vi "ManageDrive.vi"(8 "error in (no error)":errorcluster, 11 "config":T1) -> (0 "error out":errorcluster, 1 "free disk space":dbl, 2 "streams deleted":i32, 3 "files deleted":i32)   [LabVIEW 2017, in "FileManager.lvlib"]
uses:
  <vilib>/addons/InsightCM/Devices/Shared/Common/FileManager/FileManager.lvlib
  <vilib>/addons/InsightCM/Devices/Shared/Common/FileManager/controls/config.ctl
panel:
  out "config out":T1
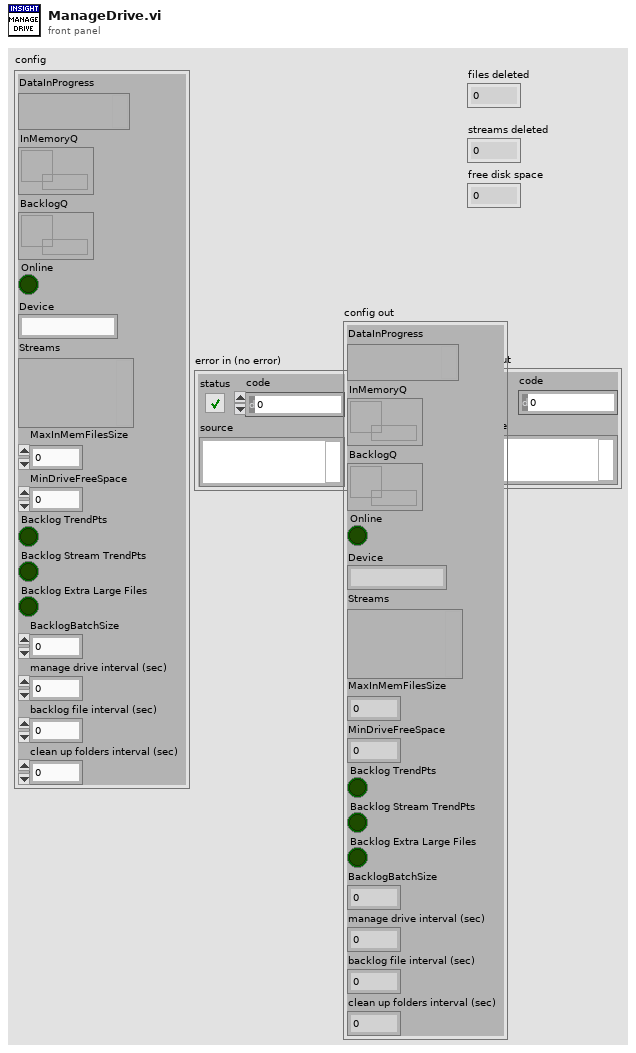
[diagram p1: front panel]
types:
  T1 = typedef "FileManager.lvlib/config.ctl" = cluster{"DataInProgress":variant, "InMemoryQ":refnum<queue>, "BacklogQ":refnum<queue>, "Online":bool, "Device":string, "Streams":variant, "MaxInMemFilesSize":i32, "MinDriveFreeSpace":i32, "Backlog TrendPts":bool, "Backlog Stream TrendPts":bool, "Backlog Extra Large Files":bool, "BacklogBatchSize":i32, "manage drive interval (sec)":dbl, "backlog file interval (sec)":dbl, "clean up folders interval (sec)":dbl}
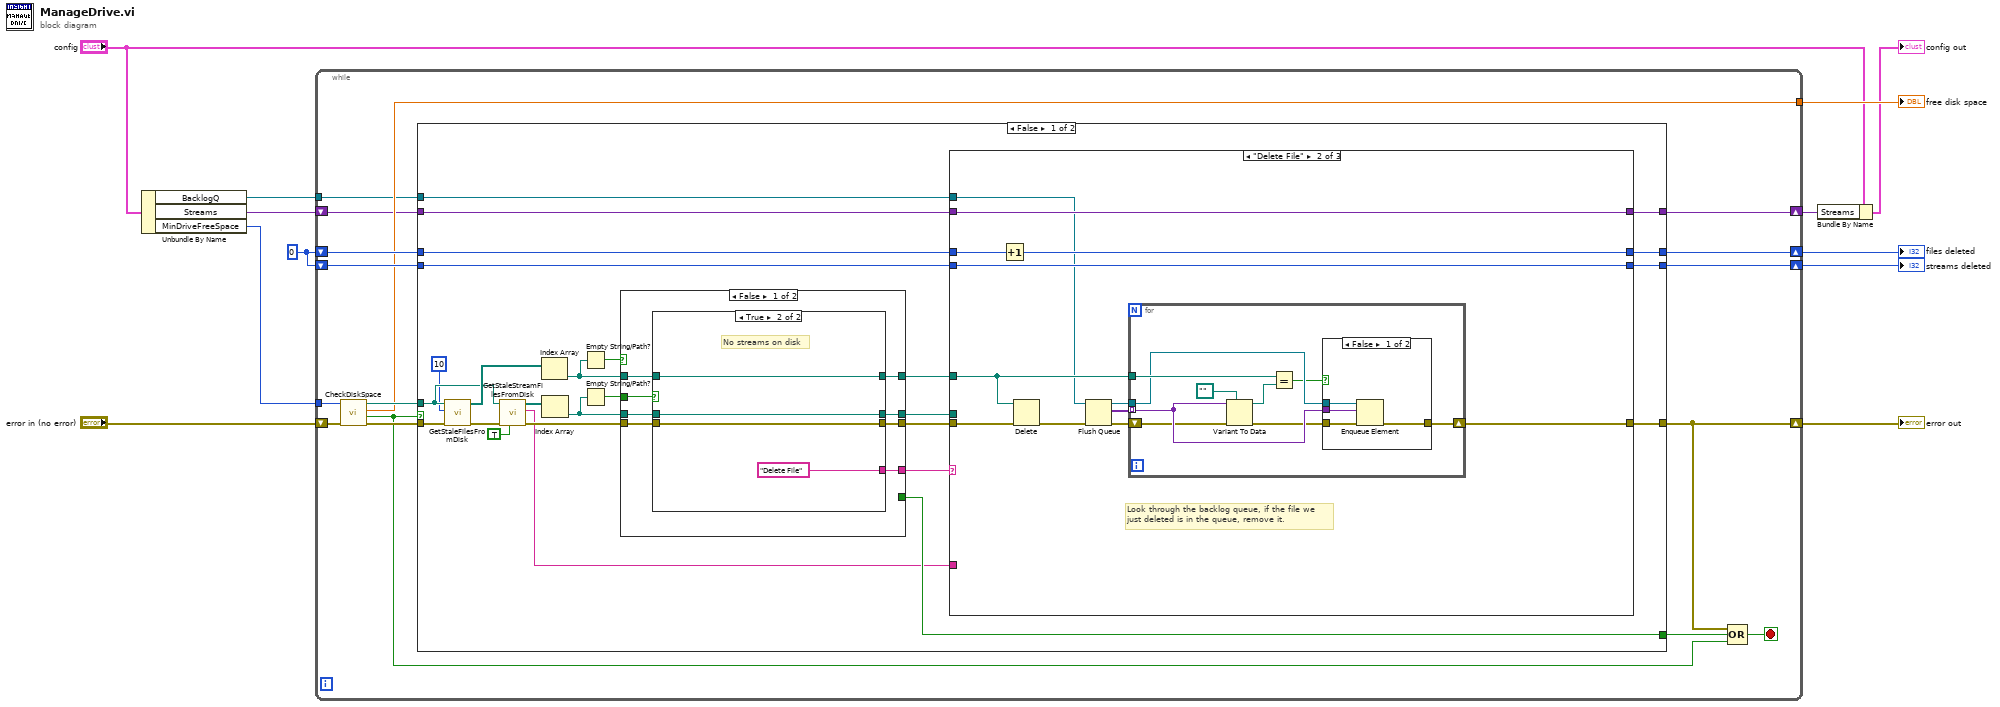
[diagram p0: block diagram]
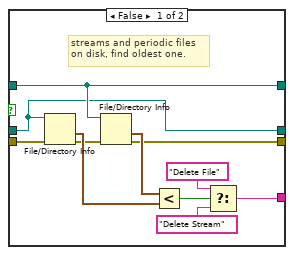
[diagram p2: hidden frame]
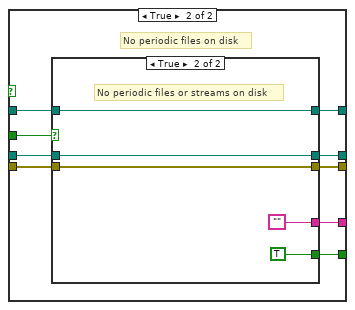
[diagram p3: hidden frame]
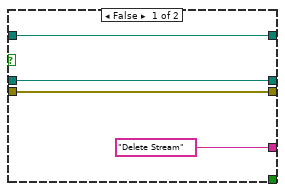
[diagram p4: hidden frame]
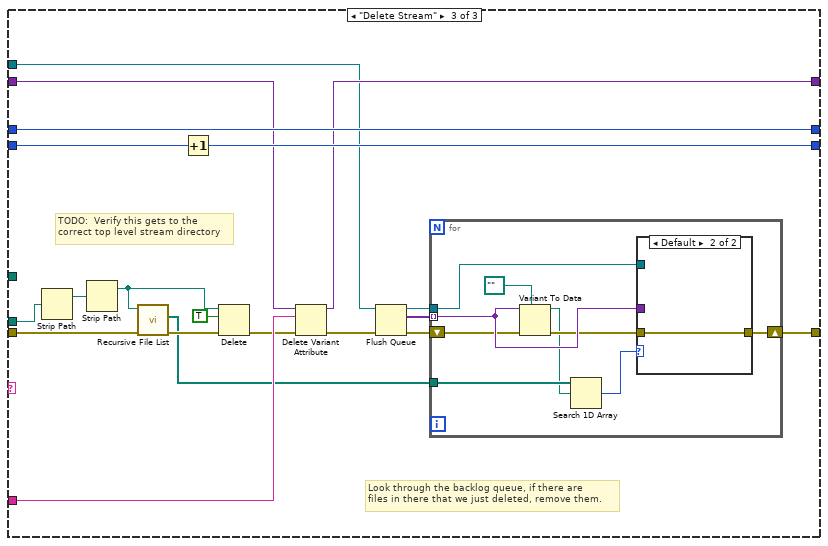
[diagram p7: hidden frame]
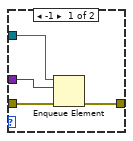
[diagram p8: hidden frame]
diagram:
  w11 = 0 ("files deleted")
  n1 = Unbundle By Name("config") -> ("BacklogQ"=w1:refnum<queue>, "Streams"=w5:variant, "MinDriveFreeSpace"=w6:i32)
  n2 = while {
    shift-right: [w18] -> w12
    shift-left: "error in (no error)" -> [w24]
    shift-right: [w25] -> w8
    shift-left: w11 -> [w27]
    shift-right: [w26] -> w9
    shift-left: w11 -> [w28]
    tunnel: w6 -> [w23]
    tunnel: [w16] -> w7
    shift-right: [w15] -> w3
    shift-left: w5 -> [w14]
    tunnel: w1 -> [w13]
    stop <- w17 stop-if-true
    n3 = call <vilib>:"CheckDiskSpace.vi"("error in (no error)"=w24, "minimum free disk space"=w23) -> ("error out"=w21:errorcluster, "available disk space"=w20:bool, "free disk space"=w16:dbl, "data directory"=w22:path)  [unwired: 6 in]
    n4 = case shown="False" w20 {
      tunnel: w21 -> [w36 w163]
      tunnel: w22 -> [w33 _]
      tunnel: w28 -> [w52 w161]
      tunnel: w27 -> [w51 w162]
      tunnel: [w50 w161] -> w26
      tunnel: [w49 w162] -> w25
      tunnel: [w48 w163] -> w18
      tunnel: [w39 _] -> w19
      tunnel: w14 -> [w38 w160]
      tunnel: [w31 w160] -> w15
      tunnel: w13 -> [w29 _]
      frame False {
        n5 = call <vilib>:"GetStaleFilesFromDisk.vi"("error in (no error)"=w36, "BacklogBatchSize"=10, "data directory"=w33) -> ("error out"=w35:errorcluster, "file paths"=w53:path[])  [unwired: 6 in, 1 out]
        n6 = call <vilib>:"GetStaleStreamFilesFromDisk.vi"("must contain block 0"=TRUE ("complete stream only"), "error in (no error)"=w35, "data directory"=w33) -> ("error out"=w34:errorcluster, "stream id"=w32:string, "file paths"=w37:path[])  [unwired: 4 in, 2 out]
        n7 = Index Array(array=w53) -> (element=w44:path)  [unwired: 1 in]
        n8 = Index Array(array=w37) -> (element=w45:path)  [unwired: 1 in]
        n9 = Empty String/Path?(string/path=w44) -> (empty?=w47:bool)
        n10 = Empty String/Path?(string/path=w45) -> (empty?=w46:bool)
        n11 = case shown="False" w47 {
          tunnel: w46 -> [w62 w86]
          tunnel: w34 -> [w59 w81]
          tunnel: w45 -> [w61 w82]
          tunnel: w44 -> [w60 w83]
          tunnel: [w58 w80] -> w43
          tunnel: [w57 w78] -> w42
          tunnel: [w56 w85] -> w41
          tunnel: [w55 w79] -> w40
          tunnel: [_ w84] -> w39
          frame False {
            n12 = case shown="True" w62 {
              tunnel: w61 -> [w65 w77]
              tunnel: w60 -> [w67 w76]
              tunnel: w59 -> [w71 w75]
              tunnel: [w67 w76] -> w58
              tunnel: [w63 w75] -> w57
              tunnel: [w66 "Delete File"] -> w56
              tunnel: [w65 w77] -> w55
              frame False {
                # "streams and periodic files \non disk, find oldest one."
                n13 = File/Directory Info(path=w65, error in=w71) -> (last mod=w72:timestamp, error out=w64:errorcluster)  [unwired: 5 out]
                n14 = File/Directory Info(path=w67, error in=w64) -> (last mod=w73:timestamp, error out=w63:errorcluster)  [unwired: 5 out]
                n15 = Less?(x=w73, y=w72) -> (x < y?=w70:bool)
                n16 = Select(t="Delete File", s=w70, f="Delete Stream") -> (s? t:f=w66:string)
              }
              frame True {
                # "No streams on disk"
              }
            }
          }
          frame True {
            # "No periodic files on disk"
            n17 = case shown="True" w86 {
              tunnel: ["Delete Stream" ""] -> w85
              tunnel: [_ TRUE] -> w84
              tunnel: w83 -> [w89 w94]
              tunnel: w82 -> [w88 w93]
              tunnel: w81 -> [w87 w92]
              tunnel: [w89 w94] -> w80
              tunnel: [w88 w93] -> w79
              tunnel: [w87 w92] -> w78
              frame False {
              }
              frame True {
                # "No periodic files or streams on disk"
              }
            }
          }
        }
        n18 = case shown="\"Delete File\"" w41 {
          tunnel: w43 -> [_ w105 _]
          tunnel: [w97 w104 w136] -> w48
          tunnel: w42 -> [w97 w111 w129]
          tunnel: w40 -> [_ _ w145]
          tunnel: w52 -> [w99 w110 w143]
          tunnel: w51 -> [w98 w108 w141]
          tunnel: [w99 w109 w143] -> w50
          tunnel: [w98 w108 w140] -> w49
          tunnel: w38 -> [w96 w102 w134]
          tunnel: w32 -> [_ _ w133]
          tunnel: [w96 w102 w132] -> w31
          tunnel: w29 -> [_ w101 w127]
          frame Default {
          }
          frame "Delete File" {
            # "Look through the backlog queue, if the file we\njust deleted is in the queue, remove it."
            n19 = Increment(x=w110) -> (x+1=w109:i32)
            n20 = Delete(path (use dialog)=w105, error in=w111) -> (error out=w100:errorcluster)  [unwired: 3 in, 2 out]
            n21 = Flush Queue(queue=w101, error in (no error)=w100) -> (queue out=w103:refnum<queue>, remaining elements=w107:variant[], error out=w106:errorcluster)
            n22 = for {
              tunnel: w107 -> [w114] mode=indexing
              tunnel: w105 -> [w120]
              shift-right: [w119] -> w104
              shift-left: w106 -> [w113]
              tunnel: w103 -> [w118]
              n23 = Variant To Data(error in=w113, type=path "", Variant=w114) -> (data=w115:path, error out=w112:errorcluster)
              n24 = Equal?(x=w120, y=w115) -> (x = y?=w117:bool)
              n25 = case shown="False" w117 {
                tunnel: w112 -> [w124 w125]
                tunnel: [w123 w125] -> w119
                tunnel: w114 -> [w122 _]
                tunnel: w118 -> [w121 _]
                frame False {
                  n26 = Enqueue Element(queue=w121, element=w122, error in (no error)=w124) -> (error out=w123:errorcluster)  [unwired: 1 in, 2 out]
                }
                frame True {
                }
              }
            }
          }
          frame "Delete Stream" {
            # "TODO:  Verify this gets to the\ncorrect top level stream directory"
            # "Look through the backlog queue, if there are \nfiles in there that we just deleted, remove them."
            n27 = Strip Path(path=w145) -> (stripped path=w144:path)  [unwired: 1 out]
            n28 = Strip Path(path=w144) -> (stripped path=w130:path)  [unwired: 1 out]
            n29 = call <vilib>:"Recursive File List.vi"("error in (no error)"=w129, "Folder Path"=w130) -> ("error out"=w128:errorcluster, "All Files in Dir"=w126:path[])  [unwired: 5 in, 3 out]
            n30 = Increment(x=w141) -> (x+1=w140:i32)
            n31 = Delete(path (use dialog)=w130, entire hierarchy (F)=TRUE, error in=w128) -> (error out=w131:errorcluster)  [unwired: 2 in, 2 out]
            n32 = Delete Variant Attribute(4:w131, 6:w133, 7:w134) -> (0:w135:errorcluster, 3:w132:variant)  [unwired: 1 out]
            n33 = Flush Queue(queue=w127, error in (no error)=w135) -> (queue out=w137:refnum<queue>, remaining elements=w139:variant[], error out=w138:errorcluster)
            n34 = for {
              tunnel: w139 -> [w151] mode=indexing
              shift-right: [w153] -> w136
              shift-left: w138 -> [w150]
              tunnel: w137 -> [w154]
              tunnel: w126 -> [w148]
              n35 = Variant To Data(error in=w150, type=path "", Variant=w151) -> (data=w147:path, error out=w149:errorcluster)
              n36 = Search 1D Array(1D array=w148, element=w147) -> (index of element=w146:i32)  [unwired: 1 in]
              n37 = case shown="Default" w146 {
                tunnel: w149 -> [w158 w159]
                tunnel: w154 -> [w157 _]
                tunnel: w151 -> [w156 _]
                tunnel: [w155 w159] -> w153
                frame -1 {
                  n38 = Enqueue Element(queue=w157, element=w156, error in (no error)=w158) -> (error out=w155:errorcluster)  [unwired: 1 in, 2 out]
                }
                frame Default {
                }
              }
            }
          }
        }
      }
      frame True {
      }
    }
    n39 = Compound Arithmetic op=OR(w18, w19, w20) -> (w17:bool)
  }
  "error out" <- w12
  "files deleted" <- w9
  "streams deleted" <- w8
  "free disk space" <- w7
  n40 = Bundle By Name(cluster="config", "Streams"=w3) -> (→"config out":T1)
